vi "create.new_video.vi"(4 "videoFileDetails":T1, 6 "Optional":T2, 8 "error in":errorcluster, 9 "Labels":string[](array[string]), 10 "Properties":map{string, string}(c390)) -> (0 "error out":errorcluster, 3 "target video":refnum<class "target.video.lvclass">)   [LabVIEW 2020, in "datasources.lvlib" / "target.video.lvclass"]
uses:
  target.video.lvclass
  C:/code/labview-client/lv_src/Nominal Client/datasources/target/target.lvclass
  dataset/dataset.lvclass
  nominal types/channelConfig/channelConfig.lvclass
  target/target.lvclass/target.ctl
  target.video.lvclass/target.video.ctl
  target/properties.set.vi
  target/labels.set.vi
  target/dataset.set.vi
  target/channelConfig.set.vi
  nominal types/labels/labels.lvclass
  nominal types/properties/properties.lvclass
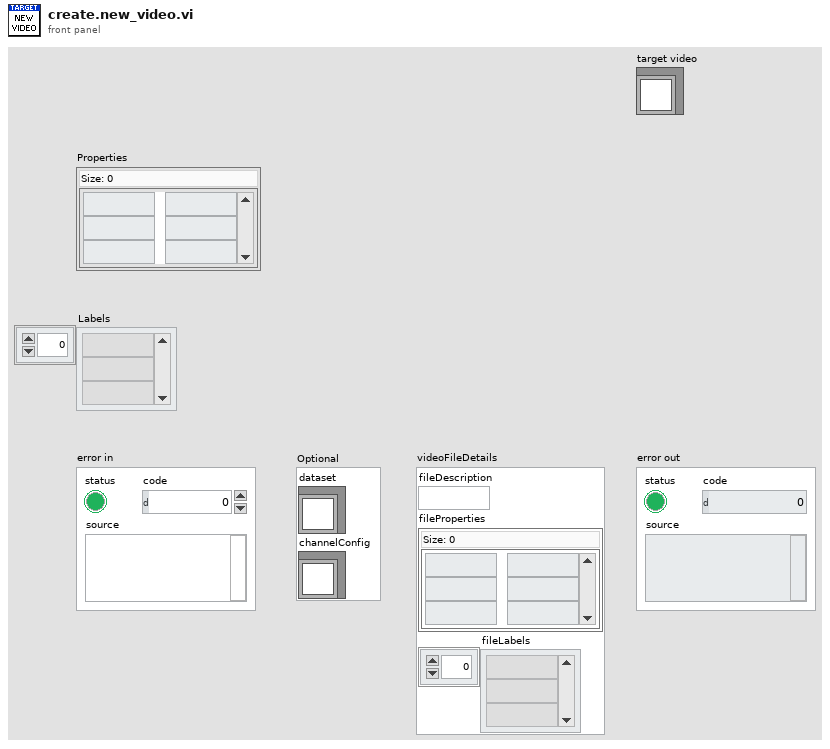
[diagram p1: front panel]
types:
  T1 = cluster{"fileDescription":string, "fileProperties":map{string, string}, "fileLabels":string[]}
  T2 = cluster{"dataset":refnum<class "dataset.lvclass">, "channelConfig":refnum<class "channelConfig.lvclass">}
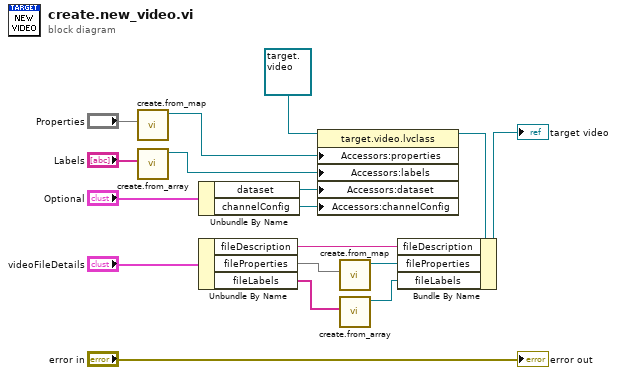
[diagram p0: block diagram]
diagram:
  n1 = call "create.from_map.vi"("properties"="Properties") -> ("properties out"=w8:refnum<class "properties.lvclass">)  [unwired: 9 in, 1 out]
  n2 = call "create.from_array.vi"("labels"="Labels") -> ("labels out"=w7:refnum<class "labels.lvclass">)  [unwired: 9 in, 1 out]
  n3 = Unbundle By Name("Optional") -> ("dataset"=w16:refnum<class "dataset.lvclass">, "channelConfig"=w15:refnum<class "channelConfig.lvclass">)
  n4 = Unbundle By Name("videoFileDetails") -> ("fileDescription"=w10:string, "fileProperties"=w4:map{string, string}, "fileLabels"=w3:string[])
  n5 = property class="target.video.lvclass"(reference=refnum<class "target.video.lvclass"> refnum ("datasources.lvlib:target.video.lvclass"), "Accessors:properties"=w8, "Accessors:labels"=w7, "Accessors:dataset"=w16, "Accessors:channelConfig"=w15) -> (reference out=w12:refnum<class "target.video.lvclass">)  [unwired: 1 in, 1 out]
  n6 = call "create.from_map.vi"("properties"=w4) -> ("properties out"=w1:refnum<class "properties.lvclass">)  [unwired: 9 in, 1 out]
  n7 = call "create.from_array.vi"("labels"=w3) -> ("labels out"=w2:refnum<class "labels.lvclass">)  [unwired: 9 in, 1 out]
  n8 = Bundle By Name(cluster=w12, "fileDescription"=w10, "fileProperties"=w1, "fileLabels"=w2) -> (→"target video":refnum<class "target.video.lvclass">)
  "error out" <- "error in"
